vi "New BrowerGuidencer.vi"(8 "error in (no error)":errorcluster, 10 "AbstractBuilder":refnum<class "AbstractBuilder.lvclass">, 11 "reference in":refnum<class "BrowerGuidencer.lvclass">) -> (0 "error out":errorcluster, 3 "reference out":refnum<class "BrowerGuidencer.lvclass">)   [LabVIEW 2015, in "BrowerGuidencer.lvclass"]
uses:
  BrowerGuidencer.lvclass
  AbstractBuilder/AbstractBuilder.lvclass
  BrowerGuidencer.lvclass/BrowerGuidencer.ctl
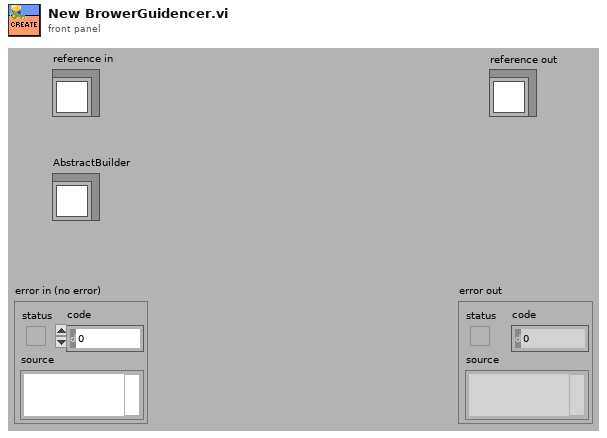
[diagram p1: front panel]
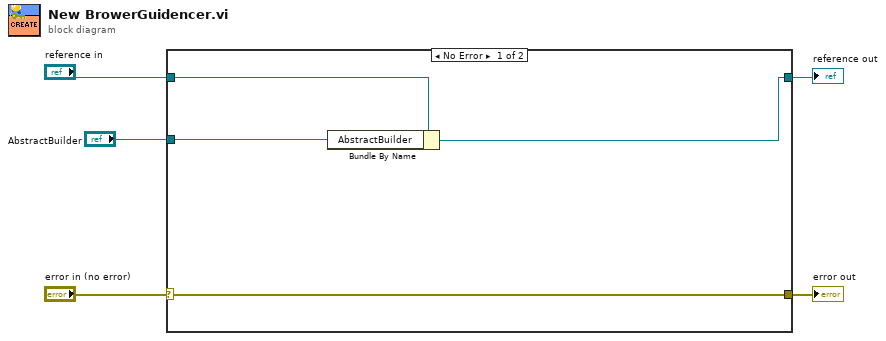
[diagram p0: block diagram]
diagram:
  n1 = case shown="No Error" "error in (no error)" {
    selector: "error in (no error)" -> [w9 w11]
    tunnel: [w9 w11] -> w4
    tunnel: "reference in" -> [w8 w10]
    tunnel: [w6 w10] -> w2
    tunnel: "AbstractBuilder" -> [w7 _]
    frame No Error {
      n2 = Bundle By Name(cluster=w8, "AbstractBuilder"=w7) -> (w6:refnum<class "BrowerGuidencer.lvclass">)
    }
    frame Error {
    }
  }
  "error out" <- w4
  "reference out" <- w2
